vi "Read Tag.vi"(8 "error in (no error)":errorcluster, 11 "Tree Data in":refnum<class "Tree Data.lvclass">) -> (0 "error out":errorcluster, 2 "Tag":string, 3 "Tree Data out":refnum<class "Tree Data.lvclass">)   [LabVIEW 2019, in "Tree Data.lvclass"]
uses:
  Tree Data.lvclass
  Tree Data.lvclass/Tree Data.ctl
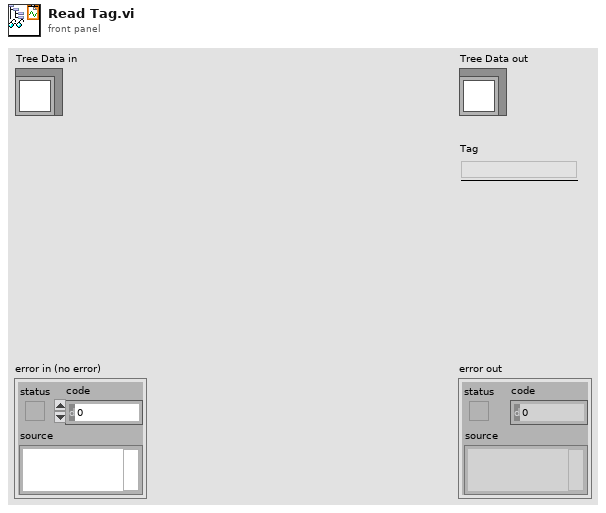
[diagram p1: front panel]
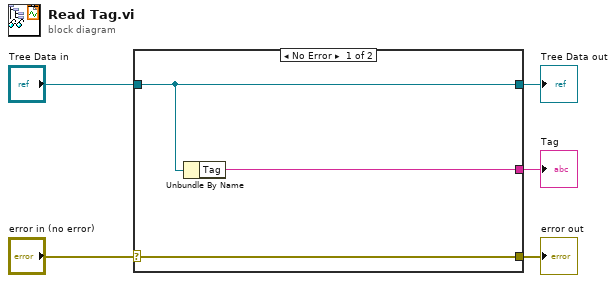
[diagram p0: block diagram]
diagram:
  n1 = case shown="No Error" "error in (no error)" {
    selector: "error in (no error)" -> [w8 w9]
    tunnel: [w8 w9] -> w4
    tunnel: [w7 w10] -> w2
    tunnel: "Tree Data in" -> [w7 w10]
    tunnel: [w6 _] -> w1
    frame No Error {
      n2 = Unbundle By Name(w7) -> ("Tag"=w6:string)
    }
    frame Error {
    }
  }
  "error out" <- w4
  "Tree Data out" <- w2
  "Tag" <- w1
